vi "rename channels.vi"(8 "error in":errorcluster, 9 "new name":string, 10 "old name":string, 11 "Scan Engine configuration in":refnum<class "Scan Engine configuration.lvclass">) -> (0 "error out":errorcluster, 3 "Scan Engine configuration out":refnum<class "Scan Engine configuration.lvclass">)   [LabVIEW 2013, in "Scan Engine configuration.lvclass"]
uses:
  Scan Engine configuration.lvclass
  Scan Engine configuration.lvclass/Scan Engine configuration.ctl
  <vilib>/NI/Tag Bus/tag/tag descriptor.lvclass/tag descriptor.ctl
  <vilib>/NI/Tag Bus/tag/read tag name.vi
  <vilib>/NI/Tag Bus/tag/tag descriptor.lvclass
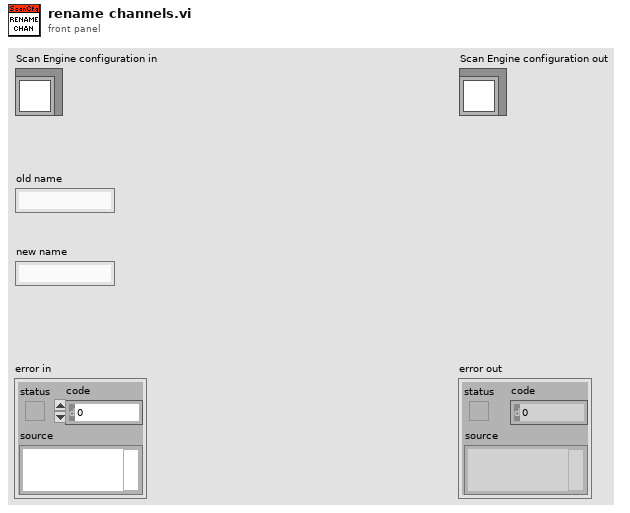
[diagram p1: front panel]
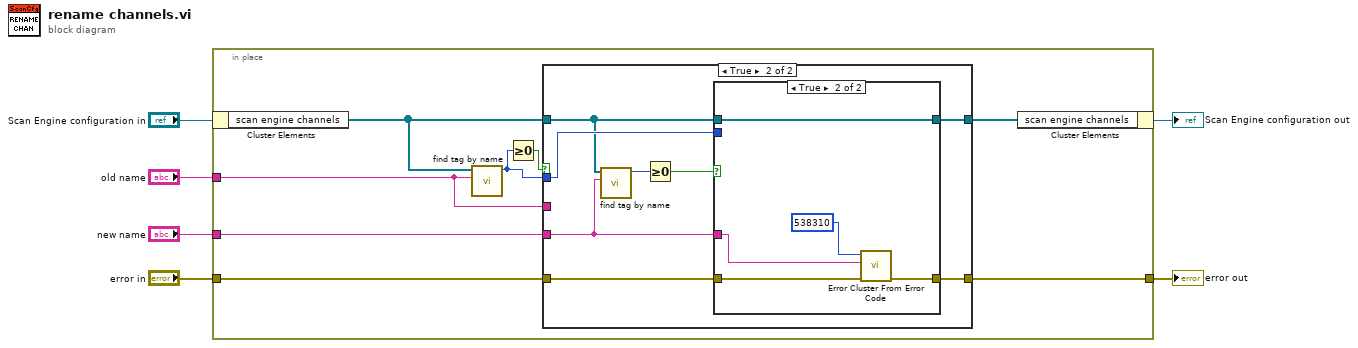
[diagram p0: block diagram]
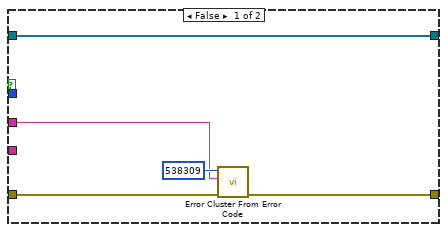
[diagram p2: hidden frame]
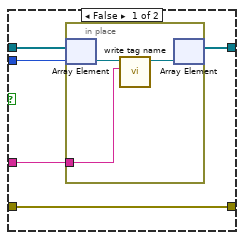
[diagram p3: hidden frame]
diagram:
  n1 = in-place {
    in-place-border: "old name" -> [w13]
    in-place-border: "new name" -> [w9]
    in-place-border: [w12] -> w1
    in-place-border: "error in" -> [w10]
    n2 = in-place-cluster #1("Scan Engine configuration in") -> ("scan engine channels"=w14:refnum<class "TBM channel.lvclass">[])
    n3 = call <vilib>:"find tag by name.vi"("name"=w13, "tags in"=w14) -> ("index"=w8:i32)  [unwired: 9 in]
    n4 = Greater Or Equal To 0?(x=w8) -> (x >= 0?=w7:bool)
    n5 = case shown="True" w7 {
      tunnel: w8 -> [_ w26]
      tunnel: w14 -> [w16 w25]
      tunnel: w13 -> [w18 _]
      tunnel: [w17 w22] -> w12
      tunnel: [w16 w27] -> w11
      tunnel: w10 -> [w15 w23]
      tunnel: w9 -> [_ w24]
      frame False {
        n6 = call <vilib>:"Error Cluster From Error Code.vi"("error in (no error)"=w15, "error message (\"\")"=w18, "error code (0)"=538309) -> ("error out"=w17:errorcluster)  [unwired: 6 in]
      }
      frame True {
        n7 = call <vilib>:"find tag by name.vi"("name"=w24, "tags in"=w25) -> ("index"=w20:i32)  [unwired: 9 in]
        n8 = Greater Or Equal To 0?(x=w20) -> (x >= 0?=w21:bool)
        n9 = case shown="True" w21 {
          tunnel: [w32 w40] -> w27
          tunnel: w26 -> [w31 _]
          tunnel: w25 -> [w30 w40]
          tunnel: w24 -> [w29 w36]
          tunnel: w23 -> [w28 w38]
          tunnel: [w28 w39] -> w22
          frame False {
            n10 = in-place {
              in-place-border: w29 -> [w33]
              n11 = in-place-array #2(w30, w31) -> (w35:refnum<class "TBM channel.lvclass">)
              n12 = call <vilib>:"write tag name.vi"("name"=w33, "system tag in"=w35) -> ("system tag out"=w34:refnum<class "TBM channel.lvclass">)  [unwired: 8 in, 1 out]
              n13 = in-place-array #2(w34) -> (w32:refnum<class "TBM channel.lvclass">[])  [unwired: 1 out]
            }
          }
          frame True {
            n14 = call <vilib>:"Error Cluster From Error Code.vi"("error in (no error)"=w38, "error message (\"\")"=w36, "error code (0)"=538310) -> ("error out"=w39:errorcluster)  [unwired: 6 in]
          }
        }
      }
    }
    n15 = in-place-cluster #1("scan engine channels"=w11) -> (→"Scan Engine configuration out":refnum<class "Scan Engine configuration.lvclass">)
  }
  "error out" <- w1
